vi "Convert R to T - SGL.vi"(8 "error in":errorcluster, 9 "R (kO)":dbl[](array[numeric])=[3.893, 10.0, 29.49], 10 "Tref (C)":dbl[](array[numeric])=[50.0, 25.0, 0.0], 11 "R":sgl caption="R (Ohms)") -> (0 "error out":errorcluster, 3 "T":sgl caption="T (degC)")   [LabVIEW 2015, in "Temperature.lvlib"]
doc: "Converts a thermistor resistance in kOhms to temperature a temperature in degrees Celsius."
uses:
  Temperature.lvlib
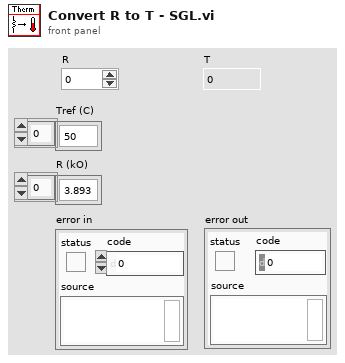
[diagram p1: front panel]
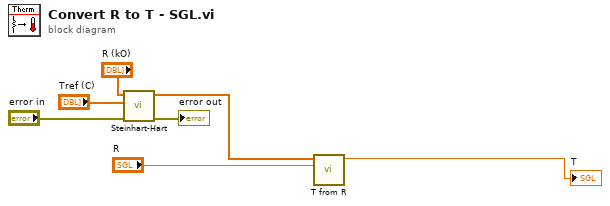
[diagram p0: block diagram]
diagram:
  n1 = call "Steinhart-Hart.vi"("error in"="error in", "Tref (C)"="Tref (C)", "R (kO)"="R (kO)") -> ("error out"=→"error out":errorcluster, "Coefficients"=w7:dbl[])  [unwired: 7 in]
  n2 = call "T from R.vi"("R"="R", "Coefficients"=w7) -> ("T"=→"T":sgl)  [unwired: 9 in]
